vi "9.vi"() -> ()   [LabVIEW 2021]
panel:
  out "Numeric":i32
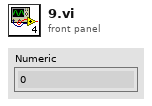
[diagram p1: front panel]
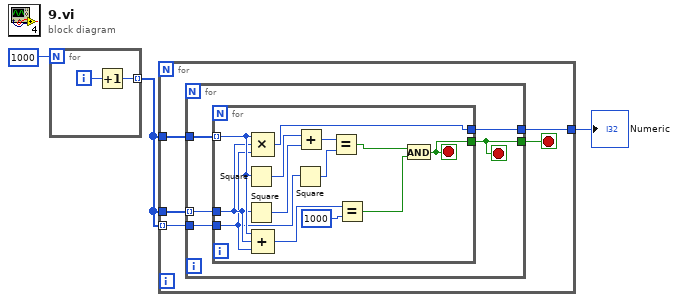
[diagram p0: block diagram]
diagram:
  n1 = for {
    N: 1000 -> [_]
    tunnel: [w4] -> w2 mode=indexing
    i -> [w5]
    n2 = Increment(x=w5) -> (x+1=w4:i32)
  }
  n3 = for {
    tunnel: w2 -> [w10]
    tunnel: w2 -> [w9]
    tunnel: w2 -> [w8] mode=indexing
    tunnel: [w7] -> w1
    stop <- w6 stop-if-true
    n4 = for {
      tunnel: w10 -> [w15]
      tunnel: w9 -> [w14] mode=indexing
      tunnel: w8 -> [w13]
      tunnel: [w12] -> w7
      tunnel: [w11] -> w6
      stop <- w11 stop-if-true
      n5 = for {
        tunnel: w15 -> [w21] mode=indexing
        tunnel: w14 -> [w20]
        tunnel: w13 -> [w19]
        tunnel: [w18] -> w12
        tunnel: [w17] -> w11
        stop <- w17 stop-if-true
        n6 = Square(x=w21) -> (x^2=w28:i32)
        n7 = Square(x=w20) -> (x^2=w27:i32)
        n8 = Compound Arithmetic op=MULTIPLY(w21, w20, w19) -> (w18:i32)
        n9 = Compound Arithmetic op=ADD(w21, w20, w19) -> (w24:i32)
        n10 = Square(x=w19) -> (x^2=w25:i32)
        n11 = Add(x=w28, y=w27) -> (x+y=w26:i32)
        n12 = Equal?(x=w26, y=w25) -> (x = y?=w16:bool)
        n13 = Equal?(x=w24, y=1000) -> (x = y?=w22:bool)
        n14 = And(x=w16, y=w22) -> (x .and. y?=w17:bool)
      }
    }
  }
  "Numeric" <- w1
